vi "Calc stop dist.vi"(8 "error in (no error)":errorcluster, 10 "Distance at speed 4":dbl=400.0, 11 "Speed":dbl) -> (0 "error out":errorcluster, 3 "Distance to start stopping":dbl=300.0)   [LabVIEW 2016]
panel:
  in  "Min dist":dbl=400.0
  out "Quadratic dist":dbl=300.0
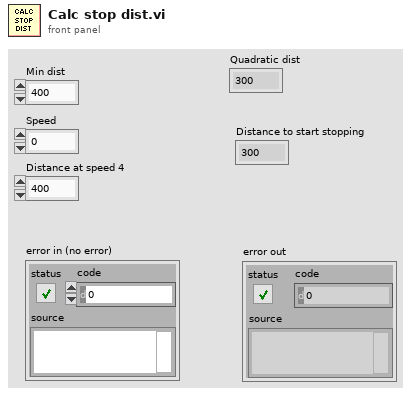
[diagram p1: front panel]
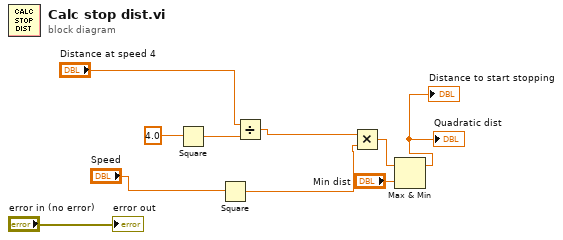
[diagram p0: block diagram]
diagram:
  n1 = Square(x=4.0) -> (x^2=w8:dbl)
  n2 = Square(x="Speed") -> (x^2=w5:dbl)
  n3 = Divide(x="Distance at speed 4", y=w8) -> (x/y=w4:dbl)
  n4 = Multiply(x=w4, y=w5) -> (x*y=w3:dbl)
  n5 = Max & Min(x=w3, y="Min dist") -> (max(x,y)=→"Distance to start stopping" →"Quadratic dist":dbl)  [unwired: 1 out]
  "error out" <- "error in (no error)"
